vi "com port send response test.vi"(0 "VISA Send port":refnum<visa-resource-name>, 1 "Wait for response msecs":u32=750, 2 "Comparison type (str in resp)":T1=enum."Get portion of string", 5 "Send text":string, 7 "Expected response":string, 11 "error in (no error)":errorcluster, 12 "PassFail_In":bool=TRUE) -> (4 "VISA Send port out":refnum<visa-resource-name>, 6 "Response":string, 10 "Log string":string, 14 "PassFail_Out":bool, 15 "error out":errorcluster)   [LabVIEW 2024]
uses:
  String/string_data_type.ctl
panel:
  in  "Wait Msecs After cmd":u32
  out "Bytes at port":u32
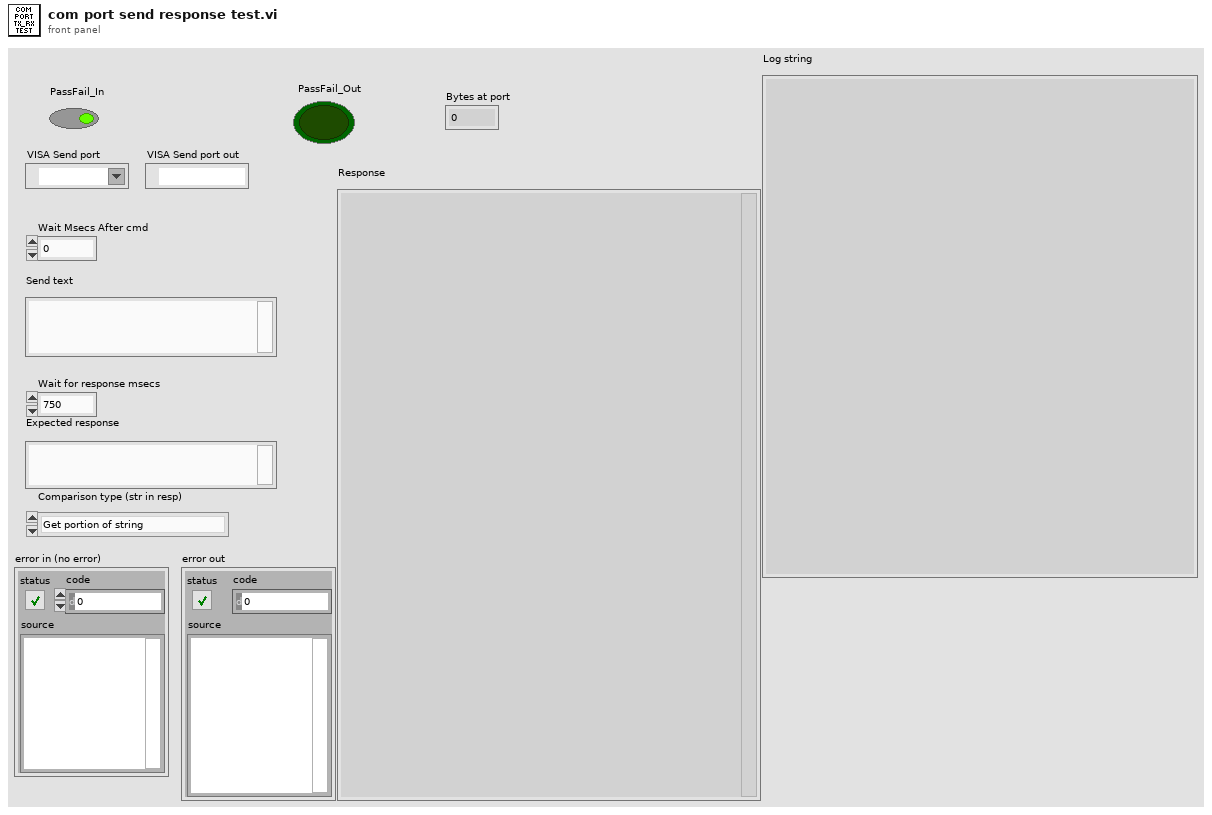
[diagram p1: front panel]
types:
  T1 = typedef "string_data_type.ctl" = enum16{"Get csv field", "Get portion of string", "Get just one line", "Get just one line with keyword", "Just Pre-Process string", "Search and replace", "Search and cut out string"}
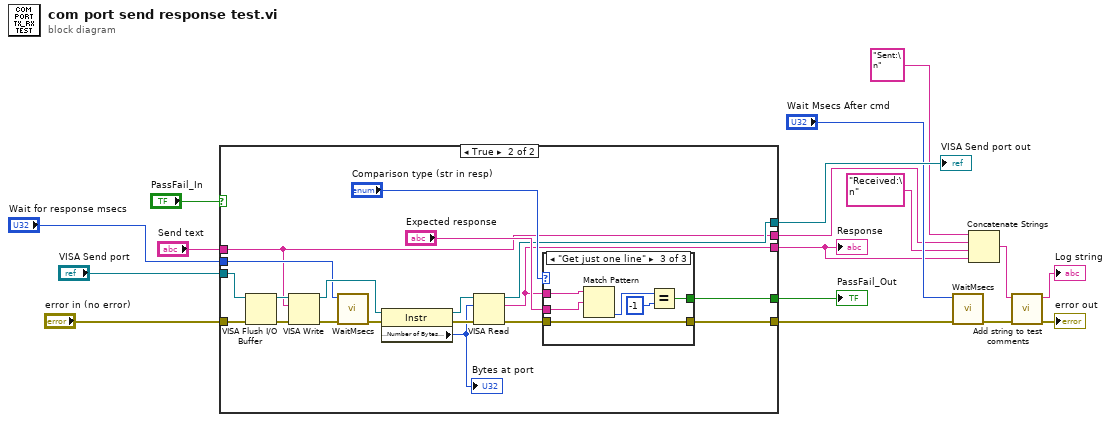
[diagram p0: block diagram]
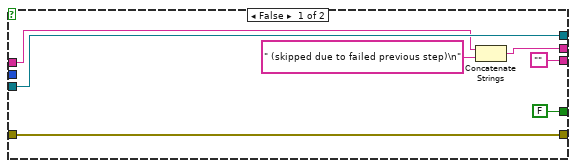
[diagram p2: hidden frame]
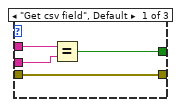
[diagram p3: hidden frame]
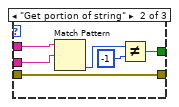
[diagram p4: hidden frame]
diagram:
  n1 = case shown="True" "PassFail_In" {
    tunnel: [FALSE w34] -> w17
    tunnel: "VISA Send port" -> [w22 w31]
    tunnel: [w23 w30] -> w11
    tunnel: "error in (no error)" -> [w23 w33]
    tunnel: [w22 w28] -> w13
    tunnel: "Wait for response msecs" -> [_ w27]
    tunnel: "Send text" -> [w21 w25]
    tunnel: ["" w26] -> w8
    tunnel: [w19 w25] -> w7
    frame False {
      n2 = Concatenate Strings(w21, " (skipped due to failed previous step)\n" ("string")) -> (w19:string)
    }
    frame True {
      n3 = VISA Flush I/O Buffer(VISA resource name=w31, error in (no error)=w33) -> (VISA resource name out=w42:refnum<visa-resource-name>, error out=w43:errorcluster)  [unwired: 1 in]
      n4 = VISA Write(VISA resource name=w42, write buffer=w25, error in (no error)=w43) -> (VISA resource name out=w29:refnum<visa-resource-name>, error out=w41:errorcluster)  [unwired: 1 out]
      n5 = call "WaitMsecs.vi"("error in (no error)"=w41, "Wait Msecs"=w27) -> ("error out"=w40:errorcluster)  [unwired: 9 in]
      n6 = property class="Instr"(reference=w29, error in=w40) -> (reference out=w37:refnum<visa-resource-name>, error out=w39:errorcluster, "Serial Settings:Number of Bytes at Serial Port"=w38:u32)
      "Bytes at port" <- w38
      n7 = VISA Read(VISA resource name=w37, byte count=w38, error in (no error)=w39) -> (VISA resource name out=w28:refnum<visa-resource-name>, read buffer=w26:string, error out=w32:errorcluster)  [unwired: 1 out]
      n8 = case shown="\"Get just one line\"" "Comparison type (str in resp)" {
        tunnel: w26 -> [w47 w53 w57]
        tunnel: w32 -> [w44 w48 w54]
        tunnel: "Expected response" -> [w46 w52 w56]
        tunnel: [w45 w49 w55] -> w34
        tunnel: [w44 w48 w54] -> w30
        frame "Get csv field", Default {
          n9 = Equal?(x=w47, y=w46) -> (x = y?=w45:bool)
        }
        frame "Get portion of string" {
          n10 = Match Pattern(string=w53, regular expression=w52) -> (offset past match=w51:i32)  [unwired: 1 in, 3 out]
          n11 = Not Equal?(x=w51, y=-1) -> (x != y?=w49:bool)
        }
        frame "Get just one line" {
          n12 = Match Pattern(string=w57, regular expression=w56) -> (offset past match=w59:i32)  [unwired: 1 in, 3 out]
          n13 = Equal?(x=w59, y=-1) -> (x = y?=w55:bool)
        }
      }
    }
  }
  "PassFail_Out" <- w17
  "VISA Send port out" <- w13
  "Response" <- w8
  n14 = call "WaitMsecs.vi"("error in (no error)"=w11, "Wait Msecs"="Wait Msecs After cmd") -> ("error out"=w3:errorcluster)  [unwired: 9 in]
  n15 = Concatenate Strings("Sent:\n" ("string"), w7, "Received:\n" ("string"), w8) -> (w4:string)
  n16 = call "Add string to test comments.vi"("error in (no error)"=w3, "Comments"=w4) -> ("error out"=→"error out":errorcluster, "concatenated string"=→"Log string":string)  [unwired: 8 in]
